vi "PWM_Wfm_Measure_v1.vi"(0 "Analysis Leg":i32, 5 "Active Leg":i32, 7 "Limits":T1={"Expected Duty Cycle"=25, "Duty Cycle Error"=1.0, "Expected Frequency"=2500.0, "Frequency Error"=0.5, "Expected Vrms"=15.8, "Vrms Error"=5.0, "Expected Vdc HIGH"=0.5, "Expected Vdc LOW"=-0.5, "Expected Vrms HIGH"=1.0} {"Expected Vrms HIGH" format="%#_13g"; "Expected Vdc LOW" format="%#_13g"; "Expected Vdc HIGH" format="%#_13g"; "Expected Vrms" format="%#_13g"; "Expected Frequency" format="%#_13g"}, 9 "Waveform":waveform(dbl)[](array[waveform]), 11 "error in (no error)":errorcluster) -> (8 "error out":errorcluster, 10 "Result (Boolean)":bool, 15 "Message":string)   [LabVIEW 2022 SP3]
uses:
  SupportVIs/Pulse Measurements 1 chan.vi
  SupportVIs/Basic Averaged DC-RMS for 1 Chan.vi
  SupportVIs/NI_MAPro.lvlib
panel:
  # "Active Legs"
  # "Inactive Legs"
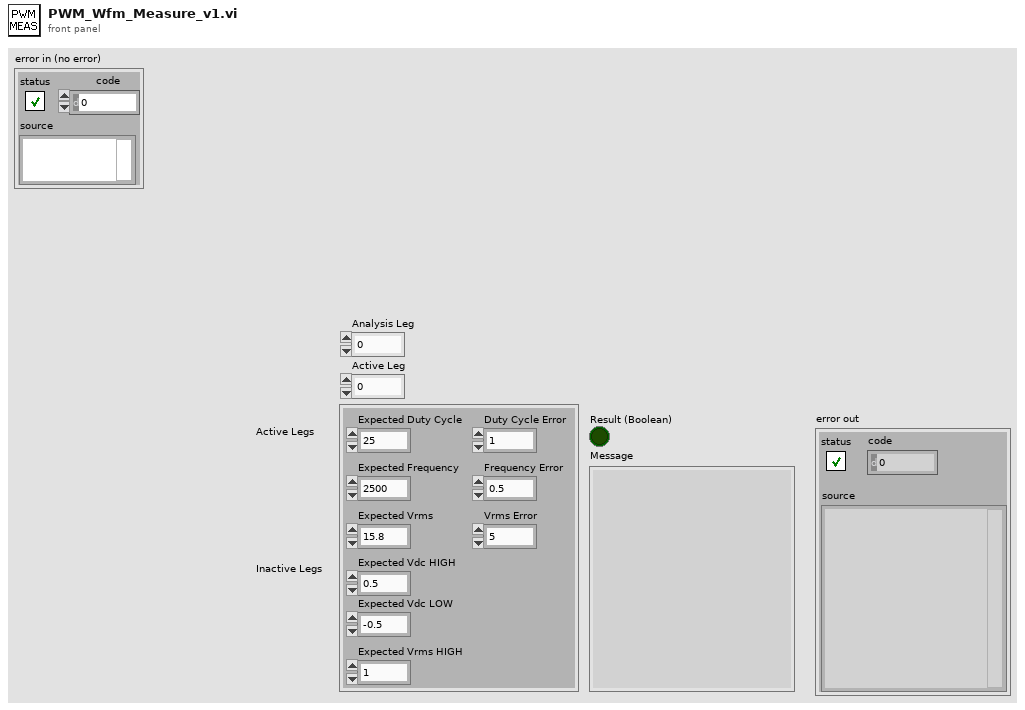
[diagram p1: front panel]
types:
  T1 = cluster{"Expected Duty Cycle":i32, "Duty Cycle Error":dbl, "Expected Frequency":dbl, "Frequency Error":dbl, "Expected Vrms":dbl, "Vrms Error":dbl, "Expected Vdc HIGH":dbl, "Expected Vdc LOW":dbl, "Expected Vrms HIGH":dbl}
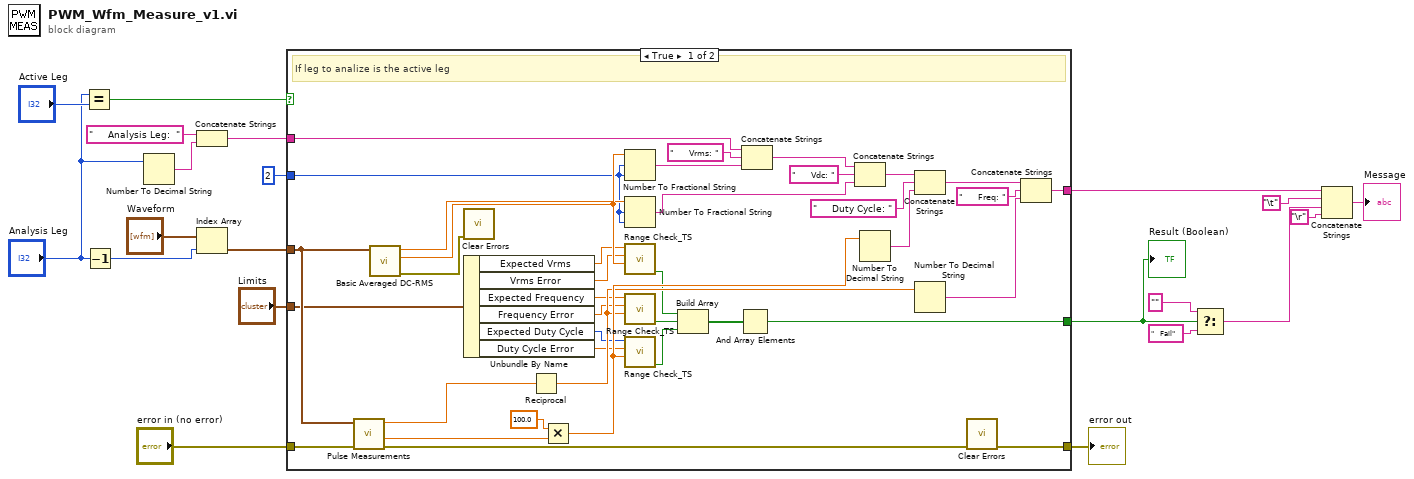
[diagram p0: block diagram]
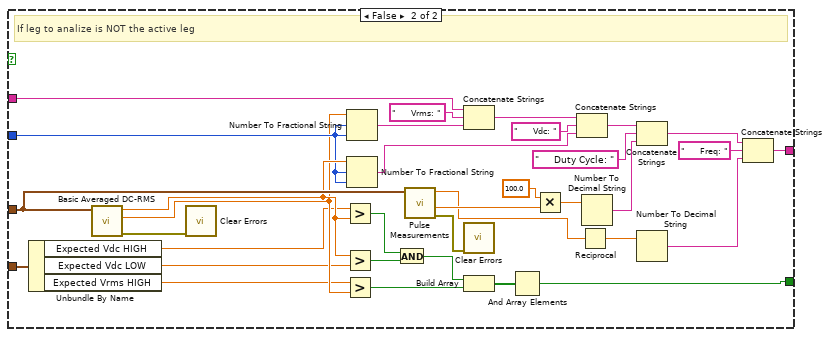
[diagram p2: hidden frame]
diagram:
  n1 = Equal?(x="Analysis Leg", y="Active Leg") -> (x = y?=w8:bool)
  n2 = Decrement(x="Analysis Leg") -> (x-1=w21:i32)
  n3 = Number To Decimal String(number="Analysis Leg") -> (decimal integer string=w4:string)  [unwired: 1 in]
  n4 = Concatenate Strings("     Analysis Leg:  ", w4) -> (w5:string)
  n5 = Index Array(array="Waveform", index=w21) -> (element=w17:waveform(dbl))
  n6 = case shown="True" w8 {
    tunnel: w17 -> [w46 w81]
    tunnel: [w40 w78] -> w13
    tunnel: [w32 w67] -> w12
    tunnel: w5 -> [w34 w69]
    tunnel: 2 -> [w31 w66]
    tunnel: "error in (no error)" -> [w30 _]
    tunnel: [w29 _] -> w2
    tunnel: "Limits" -> [w22 w63]
    frame True {
      # "If leg to analize is the active leg"
      n7 = call-poly "Pulse Measurements.vi"("error in (no error)"=w30, "signal in"=w46) -> ("error out"=w54:errorcluster, "duty cycle"=w56:dbl, "period"=w55:dbl)  [unwired: 5 in, 2 out]
      n8 = call-poly "Basic Averaged DC-RMS.vi"("signal in"=w46) -> ("error out"=w47:errorcluster, "RMS value"=w42:dbl, "DC value"=w35:dbl)  [unwired: 7 in, 1 out]
      n9 = call "Clear Errors.vi"("error in (no error)"=w47) -> ()  [unwired: 5 in, 2 out]
      n10 = Unbundle By Name(w22) -> ("Expected Vrms"=w28:dbl, "Vrms Error"=w27:dbl, "Expected Frequency"=w26:dbl, "Frequency Error"=w25:dbl, "Expected Duty Cycle"=w24:i32, "Duty Cycle Error"=w23:dbl)
      n11 = Reciprocal(x=w55) -> (1/x=w48:dbl)
      n12 = Multiply(x=100.0, y=w56) -> (x*y=w51:dbl)
      n13 = Number To Fractional String(number=w42, width (-)=w31, precision (6)=w31) -> (F-format string=w44:string)  [unwired: 1 in]
      n14 = Number To Fractional String(number=w35, width (-)=w31, precision (6)=w31) -> (F-format string=w38:string)  [unwired: 1 in]
      n15 = call "Range Check_TS.vi"("Actual Value"=w42, "Acceptable% Error"=w27, "Expected Value"=w28) -> ("Result (Boolean)"=w45:bool)  [unwired: 6 in, 2 out]
      n16 = call "Range Check_TS.vi"("Actual Value"=w48, "Acceptable% Error"=w25, "Expected Value"=w26) -> ("Result (Boolean)"=w41:bool)  [unwired: 6 in, 2 out]
      n17 = call "Range Check_TS.vi"("Actual Value"=w51, "Acceptable% Error"=w23, "Expected Value"=w24) -> ("Result (Boolean)"=w57:bool)  [unwired: 6 in, 2 out]
      n18 = Build Array(w45, w41, w57) -> (w58:bool[])
      n19 = And Array Elements(Boolean array=w58) -> (logical AND=w40:bool)
      n20 = Concatenate Strings(w34, "     Vrms: " ("string"), w44) -> (w36:string)
      n21 = Concatenate Strings(w36, "     Vdc: " ("string"), w38) -> (w33:string)
      n22 = Number To Decimal String(number=w51) -> (decimal integer string=w52:string)  [unwired: 1 in]
      n23 = Concatenate Strings(w33, "     Duty Cycle: " ("string"), w52) -> (w37:string)
      n24 = Number To Decimal String(number=w48) -> (decimal integer string=w49:string)  [unwired: 1 in]
      n25 = call "Clear Errors.vi"("error in (no error)"=w54) -> ("error out"=w29:errorcluster)  [unwired: 5 in, 1 out]
      n26 = Concatenate Strings(w37, "     Freq: " ("string"), w49) -> (w32:string)
    }
    frame False {
      # "If leg to analize is NOT the active leg"
      n27 = Unbundle By Name(w63) -> ("Expected Vdc HIGH"=w62:dbl, "Expected Vdc LOW"=w60:dbl, "Expected Vrms HIGH"=w61:dbl)
      n28 = call-poly "Basic Averaged DC-RMS.vi"("signal in"=w81) -> ("error out"=w82:errorcluster, "RMS value"=w65:dbl, "DC value"=w70:dbl)  [unwired: 7 in, 1 out]
      n29 = call "Clear Errors.vi"("error in (no error)"=w82) -> ()  [unwired: 5 in, 2 out]
      n30 = Greater?(x=w62, y=w70) -> (0:w73:bool)
      n31 = Greater?(x=w70, y=w60) -> (0:w72:bool)
      n32 = Greater?(x=w61, y=w65) -> (0:w64:bool)
      n33 = Number To Fractional String(number=w65, width (-)=w66, precision (6)=w66) -> (F-format string=w80:string)  [unwired: 1 in]
      n34 = Number To Fractional String(number=w70, width (-)=w66, precision (6)=w66) -> (F-format string=w76:string)  [unwired: 1 in]
      n35 = And(x=w73, y=w72) -> (x .and. y?=w71:bool)
      n36 = call-poly "Pulse Measurements.vi"("signal in"=w81) -> ("error out"=w89:errorcluster, "duty cycle"=w91:dbl, "period"=w90:dbl)  [unwired: 6 in, 2 out]
      n37 = Concatenate Strings(w69, "     Vrms: " ("string"), w80) -> (w74:string)
      n38 = call "Clear Errors.vi"("error in (no error)"=w89) -> ()  [unwired: 5 in, 2 out]
      n39 = Build Array(w71, w64) -> (w92:bool[])
      n40 = And Array Elements(Boolean array=w92) -> (logical AND=w78:bool)
      n41 = Multiply(x=100.0, y=w91) -> (x*y=w86:dbl)
      n42 = Concatenate Strings(w74, "     Vdc: " ("string"), w76) -> (w68:string)
      n43 = Reciprocal(x=w90) -> (1/x=w83:dbl)
      n44 = Number To Decimal String(number=w86) -> (decimal integer string=w87:string)  [unwired: 1 in]
      n45 = Concatenate Strings(w68, "     Duty Cycle: " ("string"), w87) -> (w75:string)
      n46 = Number To Decimal String(number=w83) -> (decimal integer string=w84:string)  [unwired: 1 in]
      n47 = Concatenate Strings(w75, "     Freq: " ("string"), w84) -> (w67:string)
    }
  }
  "Result (Boolean)" <- w13
  "error out" <- w2
  n48 = Select(t="" ("string"), s=w13, f="   Fail" ("string")) -> (s? t:f=w14:string)
  n49 = Concatenate Strings(w12, "\t", w14, "\r") -> (→"Message":string)
